vi "Send Send Direct Message.vi"(8 "error in (no error)":errorcluster, 10 "Message":T1, 11 "Chat Window UI Controller in":refnum<class "Chat Window UI Controller.lvclass">) -> (0 "error out":errorcluster, 3 "Chat Window UI Controller out":refnum<class "Chat Window UI Controller.lvclass">)   [LabVIEW 2015, in "Chat Window UI Controller.lvlib" / "Chat Window UI Controller.lvclass"]
uses:
  Chat Window UI Controller.lvclass
  Chat Window UI Controller Messages/Direct Message Msg/Direct Message Msg.lvclass
  <vilib>/ActorFramework/Actor/Actor.lvclass
  Controls/Message Control.ctl
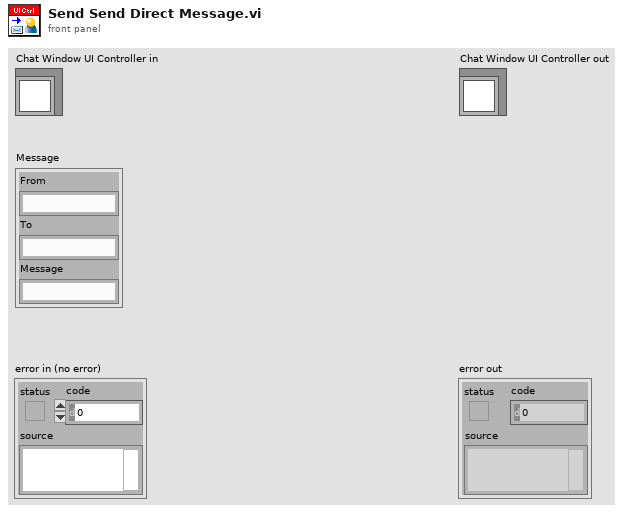
[diagram p1: front panel]
types:
  T1 = typedef "Message Control.ctl" = cluster{"From":string, "To":string, "Message":string}
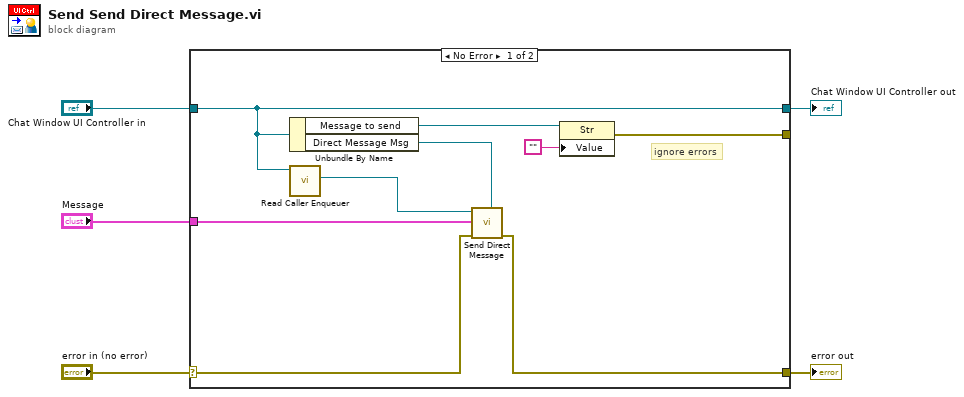
[diagram p0: block diagram]
diagram:
  n1 = case shown="No Error" "error in (no error)" {
    selector: "error in (no error)" -> [w11 w16]
    tunnel: [w10 w16] -> w4
    tunnel: [w13 w15] -> w2
    tunnel: "Chat Window UI Controller in" -> [w13 w15]
    tunnel: "Message" -> [w9 _]
    tunnel: [w6 _] -> _
    frame No Error {
      # "ignore errors"
      n2 = Unbundle By Name(w13) -> ("Message to send"=w8:refnum<vi>, "Direct Message Msg"=w14:refnum<class "Direct Message Msg.lvclass">)
      n3 = call <vilib>:"Read Caller Enqueuer.vi"("Actor"=w13) -> ("Caller Enqueuer"=w12:refnum<class "Message Enqueuer.lvclass">)  [unwired: 10 in]
      n4 = call "Send Direct Message.vi"("Message Type"=w14, "error in (no error)"=w11, "Message"=w9, "Message Enqueuer"=w12) -> ("error out"=w10:errorcluster)  [unwired: 6 in, 1 out]
      n5 = property class="Str"(reference=w8, "Value"="") -> (error out=w6:errorcluster)  [unwired: 1 in, 1 out]
    }
    frame Error {
    }
  }
  "error out" <- w4
  "Chat Window UI Controller out" <- w2
